vi "InclinometerTest.vi"() -> ()   [LabVIEW 2016]
uses:
  Telemetry/TelemetryFields.ctl
  <vilib>/rvi/Emulation/niFpgaGetClockAttributes.vi
  <vilib>/rvi/Emulation/niFpgaSctlEmulationGetInTimedLoop.vi
  <vilib>/rvi/Emulation/niFpgaEmulationReportErrorSimple.vi
  <vilib>/rvi/Emulation/niFpgaEmulationIsFPGAContextNoSignature.vi
  <vilib>/rvi/DataTransferAndStorage/Container/Common/niFpgaContainerGetUniqueNameForEmu.vi
  <vilib>/rvi/Memory/Memory_Emulation/niFpgaMemoryEmulationCacheClearOnFirstRun.vi
  <vilib>/rvi/Memory/Memory_Emulation/nirvimemoryEmulationManagerCache_MakeExclusive.vi
  <vilib>/rvi/Memory/Memory_Emulation/niFpgaMemoryEmulationValidateCache.vi
  <vilib>/rvi/Memory/Memory_Emulation/nirvimemoryEmulationManagerCache_InsertValue.vi
  <vilib>/Utility/error.llb/Clear Errors.vi
  <vilib>/rvi/Memory/Memory_Emulation/nirvimemoryEmulationManagerCache_ReleaseExclusive.vi
  <vilib>/rvi/Memory/Memory_Emulation/nirvimemoryEmulationManagerCache_GetValue.vi
  <vilib>/rvi/Memory/Memory_Emulation/nirvimemoryEmulationManagerCache_SetValue.vi
  <vilib>/rvi/Emulation/niFpgaProcessEmulError.vi
  <vilib>/rvi/Emulation/niFpgaCriticalErrorInLSC.vi
  <vilib>/rvi/DataTransferAndStorage/Container/XNode/niFpgaContainer.xnode
  <vilib>/rvi/DataTransferAndStorage/Register/Emulation/niFpgaRegisterEmulation.vi
panel:
  out "InclinometerTimestamp":u64
  out "InclinometerRxFrames":u64
  out "InclinometerTxFrames":u64
  out "InclinometerRxBytes":u64
  out "InclinometerTxBytes":u64
  out "InclinometerAngle":u32
  out "InclinometerErrorCodes":u8
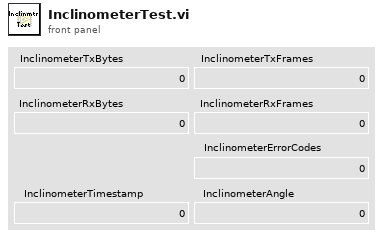
[diagram p1: front panel]
types:
  T1 = typedef "TelemetryFields.ctl" = enum16{"InclinometerErrorCode", "InclinometerTxBytes", "InclinometerRxBytes", "InclinometerTxFrames", "InclinometerRxFrames", "InclinometerTimestamp", "InclinometerAngle", "DisplacementErrorCode", "DisplacementTxBytes", "DisplacementRxBytes", "DisplacementTxFrames", "DisplacementRxFrames", "DisplacementTimestamp", "Displacement1", "Displacement2", "Displacement3", "Displacement4", "Displacement5", "Displacement6", "Displacement7", "Displacement8", "AccelerometerSampleCount", "AccelerometerTimestamp", "AccelerometerRaw1", "AccelerometerRaw2", "AccelerometerRaw3", "AccelerometerRaw4", "AccelerometerRaw5", "AccelerometerRaw6", "AccelerometerRaw7", "AccelerometerRaw8", "AccelerometerEng1", "AccelerometerEng2", "AccelerometerEng3", "AccelerometerEng4", "AccelerometerEng5", "AccelerometerEng6", "AccelerometerEng7", "AccelerometerEng8", "AngularAccelerationX", "AngularAccelerationY", "AngularAccelerationZ"}
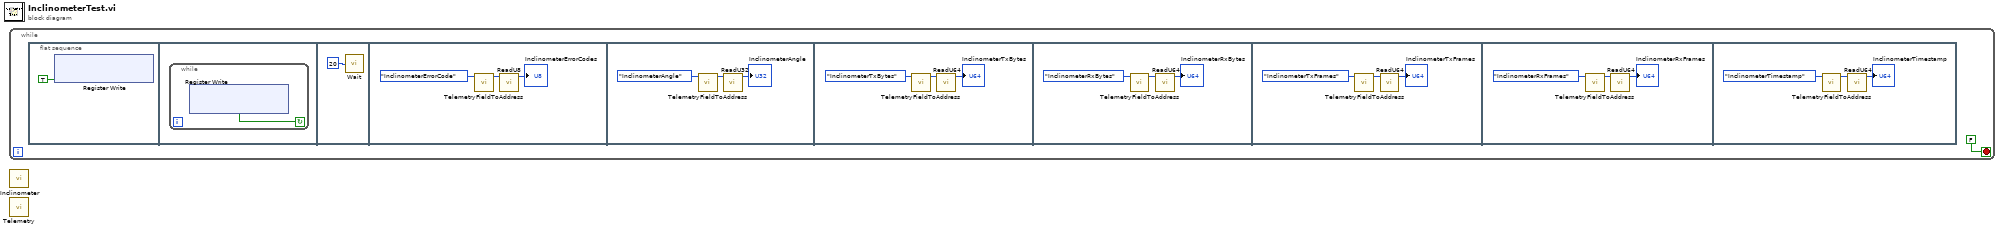
[diagram p0: block diagram]
diagram:
  n1 = while {
    stop <- FALSE stop-if-true
    n2 = flat-sequence {
      frame #0 {
        n3 = xnode ("Register Write")("Data"=TRUE) -> ()  [unwired: 1 in, 1 out]
      }
      frame #1 {
        n4 = while {
          stop <- w3 continue-if-true
          n5 = xnode ("Register Write")() -> ("Data"=w3:bool)  [unwired: 1 in, 1 out]
        }
      }
      frame #2 {
        n6 = call "Wait"("Count(mSec)"=u32 20) -> ()  [unwired: 1 out]
      }
      frame #3 {
        n7 = call "TelemetryFieldToAddress.vi"("TelemetryFields"=TelemetryFields."InclinometerErrorCode") -> ("Address"=w6:u32)  [unwired: 10 in]
        n8 = call "ReadU8.vi"("Address"=w6) -> ("Data"=→"InclinometerErrorCodes":u8)  [unwired: 10 in]
      }
      frame #4 {
        n9 = call "TelemetryFieldToAddress.vi"("TelemetryFields"=TelemetryFields."InclinometerAngle") -> ("Address"=w9:u32)  [unwired: 10 in]
        n10 = call "ReadU32.vi"("Address"=w9) -> ("Data"=→"InclinometerAngle":u32)  [unwired: 10 in]
      }
      frame #5 {
        n11 = call "TelemetryFieldToAddress.vi"("TelemetryFields"=TelemetryFields."InclinometerTxBytes") -> ("Address"=w12:u32)  [unwired: 10 in]
        n12 = call "ReadU64.vi"("Address"=w12) -> ("Data"=→"InclinometerTxBytes":u64)  [unwired: 10 in]
      }
      frame #6 {
        n13 = call "TelemetryFieldToAddress.vi"("TelemetryFields"=TelemetryFields."InclinometerRxBytes") -> ("Address"=w15:u32)  [unwired: 10 in]
        n14 = call "ReadU64.vi"("Address"=w15) -> ("Data"=→"InclinometerRxBytes":u64)  [unwired: 10 in]
      }
      frame #7 {
        n15 = call "TelemetryFieldToAddress.vi"("TelemetryFields"=TelemetryFields."InclinometerTxFrames") -> ("Address"=w18:u32)  [unwired: 10 in]
        n16 = call "ReadU64.vi"("Address"=w18) -> ("Data"=→"InclinometerTxFrames":u64)  [unwired: 10 in]
      }
      frame #8 {
        n17 = call "TelemetryFieldToAddress.vi"("TelemetryFields"=TelemetryFields."InclinometerRxFrames") -> ("Address"=w21:u32)  [unwired: 10 in]
        n18 = call "ReadU64.vi"("Address"=w21) -> ("Data"=→"InclinometerRxFrames":u64)  [unwired: 10 in]
      }
      frame #9 {
        n19 = call "TelemetryFieldToAddress.vi"("TelemetryFields"=TelemetryFields."InclinometerTimestamp") -> ("Address"=w24:u32)  [unwired: 10 in]
        n20 = call "ReadU64.vi"("Address"=w24) -> ("Data"=→"InclinometerTimestamp":u64)  [unwired: 10 in]
      }
    }
  }
  n21 = call "Inclinometer.vi"() -> ()  [unwired: 12 in]
  n22 = call "Telemetry.vi"() -> ()  [unwired: 12 in]
